vi "Synthetic_Jet_Optimisation.vi"() -> (5 "Plug in titles":string[](array[string]), 7 "Plug in values":string[](array[string]))   [LabVIEW 2011]
uses:
  Controls/SJ_Channels.ctl
  Controls/SJ_Data_Cluster.ctl
  <vilib>/Analysis/2dsp.llb/Integral Method.ctl
  Globals/Meas_global.vi
  Globals/Plug_in_data_global.vi
  <vilib>/Analysis/1siggen.llb/Ramp Pattern by Delta.vi
  <vilib>/Analysis/baseanly.llb/Scale 1D.vi
  <vilib>/Analysis/5stat.llb/RMS (DBL).vi
  <vilib>/Analysis/8numeric.llb/1D Numeric Integration.vi
  Acquisition/Data_Translation/DataTranslation_global.vi
  <vilib>/Analysis/baseanly.llb/Quick Scale 1D.vi
  <vilib>/Analysis/1siggen.llb/Ramp Pattern by Samples.vi
  <vilib>/Utility/file.llb/Write To Spreadsheet File (DBL).vi
  <vilib>/Analysis/NI_AALBase.lvlib
  <vilib>/Analysis/NI_AALPro.lvlib
panel:
  out "Target Value 2":dbl
  out "Array":dbl[][][](array[numeric])
  out "Max Amp":dbl
  out "Min Amp":dbl
  out "Sweep Frequency":dbl[](array[numeric])
  out "Last Block in Iteration?":bool
  out "Max Input Voltage _V_":dbl
  out "Sweep Size":i32
  out "Optimisation Coefficient":dbl
  out "ID Number":i32
  out "Max Number of Iterations":i32
  out "Optimisation Type":i32
  out "Target Value":dbl
  out "Phase Average?":bool
  out "Samps per cyle":i32
  out "Formation Criteria":dbl
  out "Jet Formation":bool
  out "Strouhal Number":dbl
  out "Stokes Number":dbl
  out "nu":dbl=1.55e-05
  out "Omega":dbl=1200.0
  out "Reynolds Number":dbl
  out "Charicteristic Velocity m_s":dbl
  out "Stroke Length _m_":dbl
  out "Cavity:Helmholtz:Hz":dbl=428.16291209383184
  out "LEM Velocity _ms_":dbl[](array[numeric])=[3.7049856348371377, 3.4607988115264297, 3.0653584733968287, 2.5359472607578692, 1.895702983998723, 1.1726073902466658, 0.3982632267462864, -0.3934869508418966, -1.1680398605184126, -1.8915438234131698, -2.5323782445904723, -3.062535584780142, -3.458845424238726, -3.7039871212762807, -3.787246807411894, -3.7049856348371377, -3.4607988115264297, -3.0653584733968295, -2.5359472607578692, -1.8957029839987247, -1.172607390246666, -0.3982632267462887, 0.3934869508418962, 1.1680398605184101, 1.8915438234131694, 2.53237824459047, 3.0625355847801417, 3.4588454242387248, 3.7039871212762803, 3.7872468074118935]
  out "LEM Max Velocity _ms_":dbl=3.7872475686779676
  out "LEM Phase Velocity _deg_":dbl=-258.0363282123533
  out "Phase Pressure _deg_":dbl=-169.14507601114087
  out "Phase Velocity _deg_":dbl=373.1272896341652
  out "Phase Input Voltage _deg_":dbl=8.606071626556414
  out "Phase Angle _deg_":dbl[](array[numeric])=[0.0, 12.0, 24.0, 36.0, 48.0, 60.0, 72.0, 84.0, 96.0, 108.0, 120.0, 132.0, 144.0, 156.0, 168.0, 180.0, 192.0, 204.0, 216.0, 228.0, 240.0, 252.0, 264.0, 276.0, 288.0, 300.0, 312.0, 324.0, 336.0, 348.0]
  out "Amplitude (V)":dbl=70.0
  out "Frequency (Hz)":dbl=1200.0
  out "AS Freq":dbl=36036.04
  out "Output Data Names":string[](array[string])=["Max Pressure _Pa_", "Max Velocity m_s", "Max Current _A_", "Max Displacement _m_", "Phase Displ _deg_", "Phase Pressure _deg_", "Phase Velocity _deg_", "Phase Current _deg_", "Phase Input Voltage _deg_", "LEM Max Velocity _ms_", "LEM Phase Velocity _deg_"]
  out "Input Voltage _V_":dbl[](array[numeric])=[-5.5088632433799996, -12.651031578584, -19.235618350895997, -24.9961110527, -29.670494279084004, -33.04444558276, -35.005182361704, -35.409211536216006, -34.310616683552006, -31.700640287920002, -27.711473499856005, -22.510574222680006, -16.349366000988, -9.495663135284, -2.196569584672, 5.184714435096, 12.336113665324001, 18.917564300223997, 24.689891482827996, 29.395636083331993, 32.795741589576, 34.758786092276, 35.215182844328, 34.127830748423996, 31.539748142271996, 27.582652797175996, 22.404475723135995, 16.265220463328, 9.402109185388, 2.133489422836]
  out "Pressure _Pa_":dbl[](array[numeric])=[-27.3956675953706, 95.65286233449294, 217.28142105099454, 325.3916285730047, 412.49320713856633, 477.62511872885386, 518.8812420389512, 544.5955786383588, 546.2858417945154, 525.7943338813993, 485.98446016799124, 431.53940396868336, 357.29264741860004, 257.81676584697294, 146.44897730607346, 25.39291194062997, -95.29994862668336, -216.63005998968256, -325.4638615668826, -412.65459893301875, -477.423305725176, -519.6780076017092, -543.7330519967387, -544.6659346048561, -524.568602441649, -487.2326508157636, -435.0203186855821, -361.9795522274816, -267.2741357434412, -152.01151538796677]
  out "Zeros":dbl[](array[numeric])=[1.4978743085562871, 0.2341330189017041, -0.35175473981443495, 0.0022887999999999997, -3.0068544366899315, 2.8293]
  out "Velocity m_s":dbl[](array[numeric])=[-0.006589971422005106, -0.006419643065741468, -0.009111611844261746, -0.006030326884042168, -0.004272653157727323, -0.0068849933436421745, -0.010636233235274354, -0.0035467148583991693, -0.008496862890472292, -0.005357351691532665, -0.007065956289182962, -0.006648911559621155, -0.005058171342073957, -0.008830133605031026, -0.0038751674420970687, -0.005274584307176274, 0.000979796600094568, -0.005616008146962059, -0.00729733372181674, 0.0005036149760482819, -0.004633370846616606, -0.007598533001820504, -0.005354959759266961, -0.003855515705978843, -0.005082756078867318, -0.0008163141834672163, -0.007346968606858383, -0.00413574997102441, -0.00277648312445221, -0.00052352239052674]
  out "RMS Velocity m_s":dbl=0.014914535983039488 format="%0.2f"
  out "RMS Pressure _Pa_":dbl=395.7699897259115 format="%0.2f"
  out "Max Pressure _Pa_":dbl=546.2858417945154 format="%0.2f"
  out "Max Velocity m_s":dbl=0.000979796600094568
  in  "Menu Ring":u16(ring) items=["Max Pressure _Pa_", "Input", "Max Velocity m_s"]
  out "Frequency Plot":cluster{"Sweep Frequency":dbl[], dbl[]}[](graph)
  out "Pressure Plot":cluster{dbl[], dbl[]}[](graph)=[{[0.0, 12.0, 24.0, 36.0, 48.0, 60.0, 72.0, 84.0, 96.0, 108.0, 120.0, 132.0, 144.0, 156.0, 168.0, 180.0, 192.0, 204.0, 216.0, 228.0, 240.0, 252.0, 264.0, 276.0, 288.0, 300.0, 312.0, 324.0, 336.0, 348.0], [-0.15557712257291065, -0.35728080433659803, -0.5432376920119246, -0.705921142218441, -0.8379315153272326, -0.9332160799164545, -0.9885897155857659, -1.0, -0.9689743203815658, -0.8952653536353687, -0.7826063416157439, -0.6357265029653804, -0.4617263500562873, -0.2681692905127802, -0.06203384626131485, 0.1464227586596542, 0.34838713233438734, 0.5342554516040381, 0.697273122209331, 0.8301691793748806, 0.926192371045399, 0.9816311796924717, 0.9945203893712923, 0.9638122191316959, 0.8907215601232357, 0.7789682853842954, 0.632730149899583, 0.45934997583022086, 0.26552721106968635, 0.060252384345070756]}, {[0.0, 12.0, 24.0, 36.0, 48.0, 60.0, 72.0, 84.0, 96.0, 108.0, 120.0, 132.0, 144.0, 156.0, 168.0, 180.0, 192.0, 204.0, 216.0, 228.0, 240.0, 252.0, 264.0, 276.0, 288.0, 300.0, 312.0, 324.0, 336.0, 348.0], [-0.05014896140338823, 0.1750967259562854, 0.39774309423293575, 0.5956435325215701, 0.7550867615085017, 0.8743135592895557, 0.9498346878887768, 0.9969058997564276, 1.0, 0.9624894032658751, 0.8896156974736197, 0.7899516534258018, 0.6540397353973438, 0.47194480640402603, 0.2680812243366908, 0.0464828300459258, -0.17445070206035157, -0.39655074947222896, -0.5957757581594167, -0.7553821962097238, -0.87394413180629, -0.9512932019153176, -0.9953270072140422, -0.9970346894139926, -0.9602456485390019, -0.8919005647578826, -0.7963236192550169, -0.6626193185574809, -0.4892569334498257, -0.2782636922981901]}]
  out "Velocity Plot":cluster{dbl[], dbl[]}[](graph)=[{[0.0, 12.0, 24.0, 36.0, 48.0, 60.0, 72.0, 84.0, 96.0, 108.0, 120.0, 132.0, 144.0, 156.0, 168.0, 180.0, 192.0, 204.0, 216.0, 228.0, 240.0, 252.0, 264.0, 276.0, 288.0, 300.0, 312.0, 324.0, 336.0, 348.0], [-0.15557712257291065, -0.35728080433659803, -0.5432376920119246, -0.705921142218441, -0.8379315153272326, -0.9332160799164545, -0.9885897155857659, -1.0, -0.9689743203815658, -0.8952653536353687, -0.7826063416157439, -0.6357265029653804, -0.4617263500562873, -0.2681692905127802, -0.06203384626131485, 0.1464227586596542, 0.34838713233438734, 0.5342554516040381, 0.697273122209331, 0.8301691793748806, 0.926192371045399, 0.9816311796924717, 0.9945203893712923, 0.9638122191316959, 0.8907215601232357, 0.7789682853842954, 0.632730149899583, 0.45934997583022086, 0.26552721106968635, 0.060252384345070756]}, {[0.0, 12.0, 24.0, 36.0, 48.0, 60.0, 72.0, 84.0, 96.0, 108.0, 120.0, 132.0, 144.0, 156.0, 168.0, 180.0, 192.0, 204.0, 216.0, 228.0, 240.0, 252.0, 264.0, 276.0, 288.0, 300.0, 312.0, 324.0, 336.0, 348.0], [-0.0017400427690923374, -0.0016950685794170583, -0.002405866928563968, -0.0015922719565676093, -0.001128168660507009, -0.0018179415532591603, -0.002808434141249664, -0.0009364889690996669, -0.002243546122698781, -0.0014145768585897204, -0.0018657237429983216, -0.001755605561963586, -0.0013355800662831847, -0.0023315442732039188, -0.0010232149208002786, -0.001392722622896813, 0.00025870946624789303, -0.0014828735576385352, -0.0019268175782828233, 0.00013297653986074366, -0.0012234140213805954, -0.002006347457194939, -0.0014139452830977239, -0.0010180259967302217, -0.001342071519849202, -0.00021554290622666447, -0.0019399233745421283, -0.001092020188103525, -0.0007331138596561618, -0.00013823297428152076]}, {[0.0, 12.0, 24.0, 36.0, 48.0, 60.0, 72.0, 84.0, 96.0, 108.0, 120.0, 132.0, 144.0, 156.0, 168.0, 180.0, 192.0, 204.0, 216.0, 228.0, 240.0, 252.0, 264.0, 276.0, 288.0, 300.0, 312.0, 324.0, 336.0, 348.0], [0.9782794265180274, 0.9138033477917035, 0.8093896778519208, 0.6696017951074252, 0.5005491008108334, 0.3096200089077361, 0.10515903689372944, -0.10389788964157722, -0.3084139798421589, -0.49945089918916635, -0.6686594176102914, -0.8086443108979737, -0.9132875674934984, -0.9780157749495838, -1.0, -0.9782794265180274, -0.9138033477917035, -0.8093896778519211, -0.6696017951074252, -0.5005491008108338, -0.30962000890773617, -0.10515903689373006, 0.10389788964157712, 0.3084139798421583, 0.4994508991891662, 0.6686594176102908, 0.8086443108979736, 0.9132875674934979, 0.9780157749495837, 0.9999999999999999]}]
  out "Amplitude String":string="3.5000"
  out "Frequency String":string="1200"
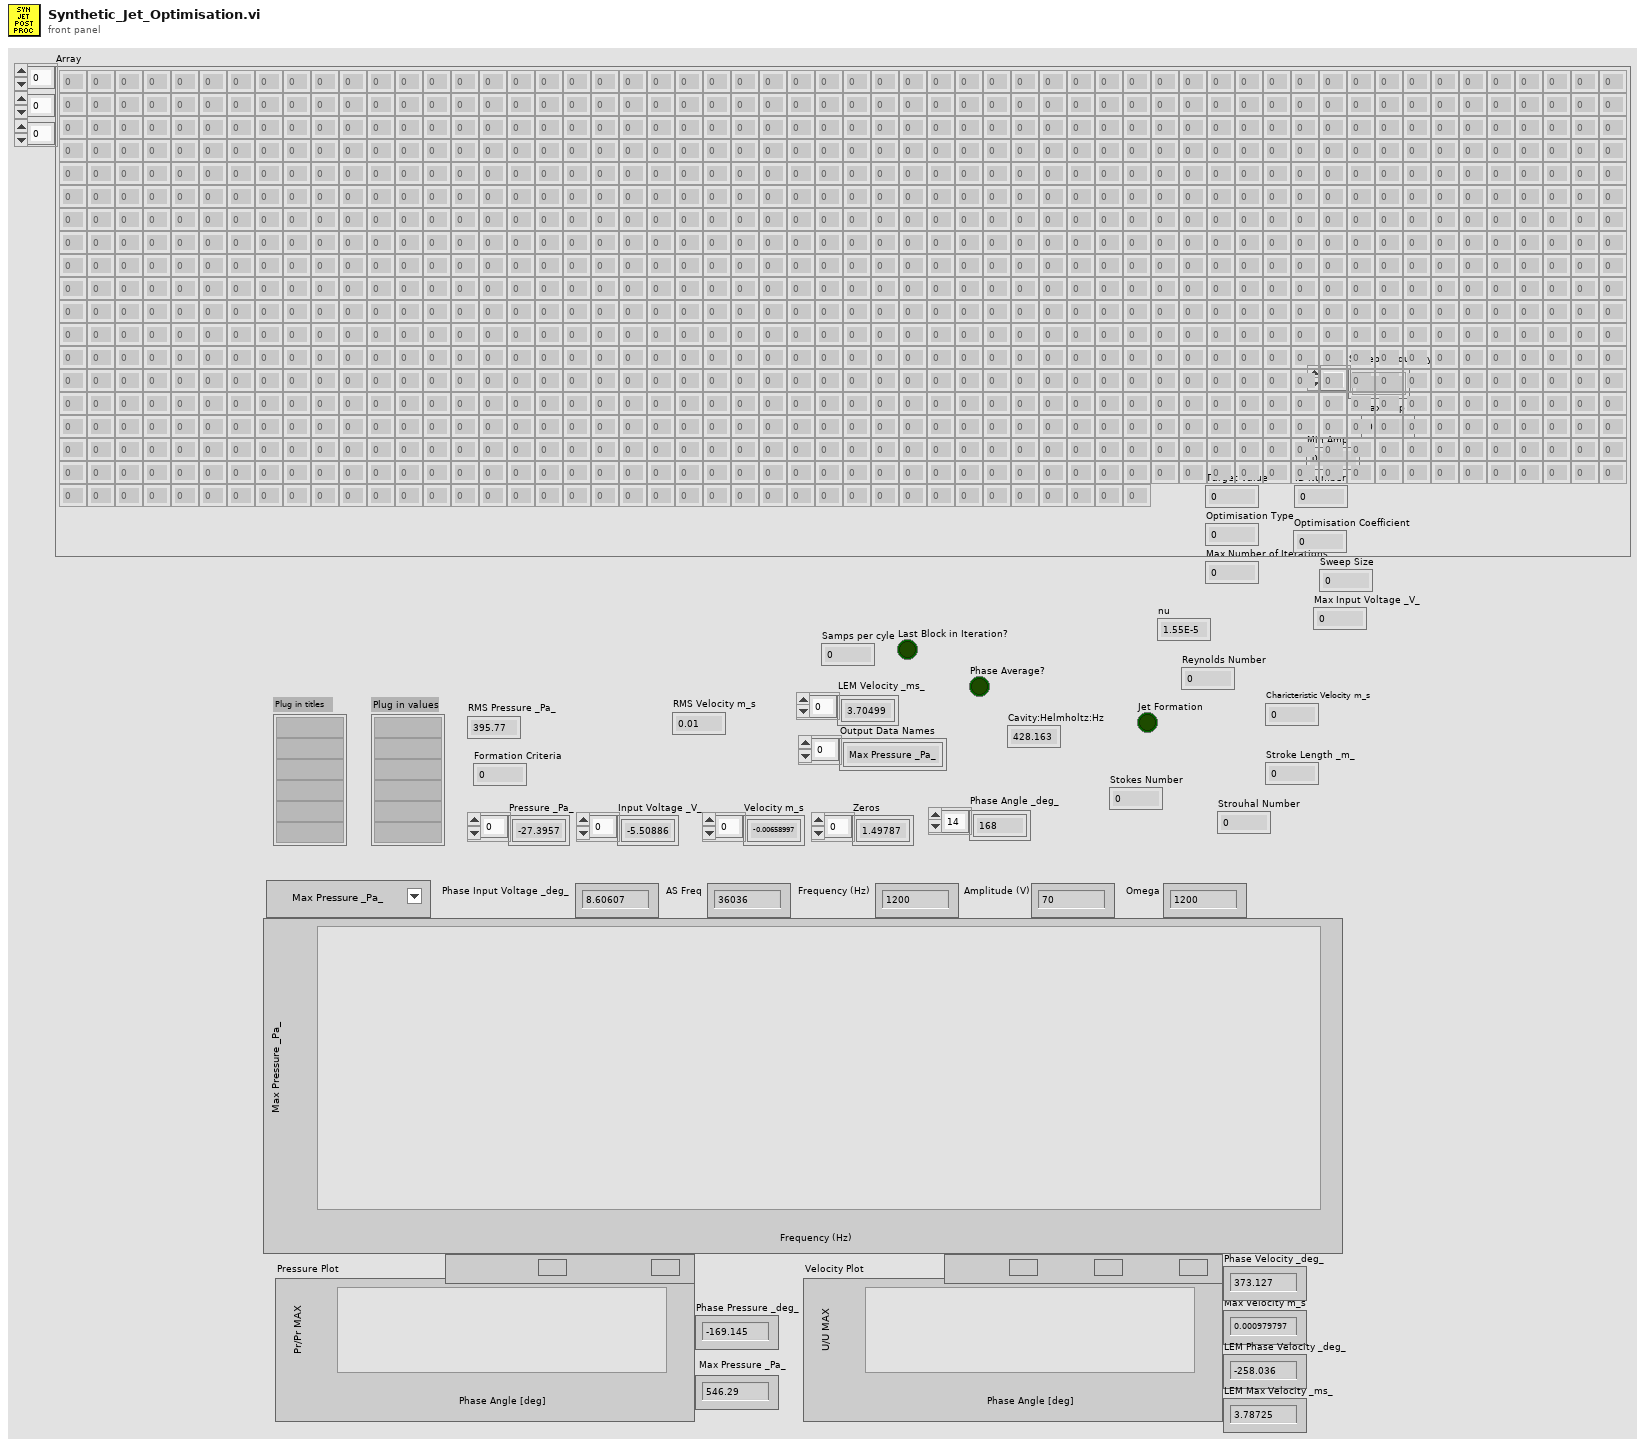
[diagram p1: front panel]
types:
  T1 = typedef "SJ_Channels.ctl" = string[]
  T2 = typedef "Analysis_info_cluster.ctl" = cluster{"Colour":u32, "Inst type":T3, "Inst name":string, "Symbol":string, "Code name":string, "Extra Info":string, "Inst Array":T4, "Index":i32, "Voltage Index":i32, "Extra Titles":string[], "Extra Values":string[]}
  T3 = typedef "Inst_type.ctl" = enum16{"Propeller anemometer", "Raw voltage", "Pressure Transducer", "Pitot-static tube", "Preston tube", "Hot wire", "Cross wire 1", "Cross wire 2", "Generic Linear", "Generic Polynomial", "Generic BackPoly", "Fast FID", "Thermocouple", "Cold wire", "Pulsed Wire", "LDA Vel", "LDA Tran time", "LDA Arr time"}
  T4 = typedef "Instrument_Array.ctl" = enum16{"PWA", "LDA", "Analogue"}
  T5 = typedef "Post_Process.ctl" = enum16{"Take New Data", "Post Process Raw Data File"}
  T6 = cluster{"Name":string, "X":dbl, "Y":dbl, "Z":dbl}[]
  T7 = typedef "SJ_Data_Cluster.ctl" = cluster{"Do":dbl, "Dc":dbl, "Ho":dbl, "Hc":dbl, "K":dbl, "beta":dbl, "Vc":dbl, "Vo":dbl}
  T8 = cluster{"R":dbl, "Mair":dbl, "T":dbl, "Patmos":dbl, "gamma":dbl}
  T9 = typedef "NI_AALPro.lvlib/Integral Method.ctl" = i32
  T10 = cluster{"Ramp Pattern":dbl[], "Y[i]=X[i]/Max|X|":dbl[]}
  T11 = cluster{"Ramp Pattern":dbl[], "Y[i]=X[i]/Max|X|":dbl[]}[]
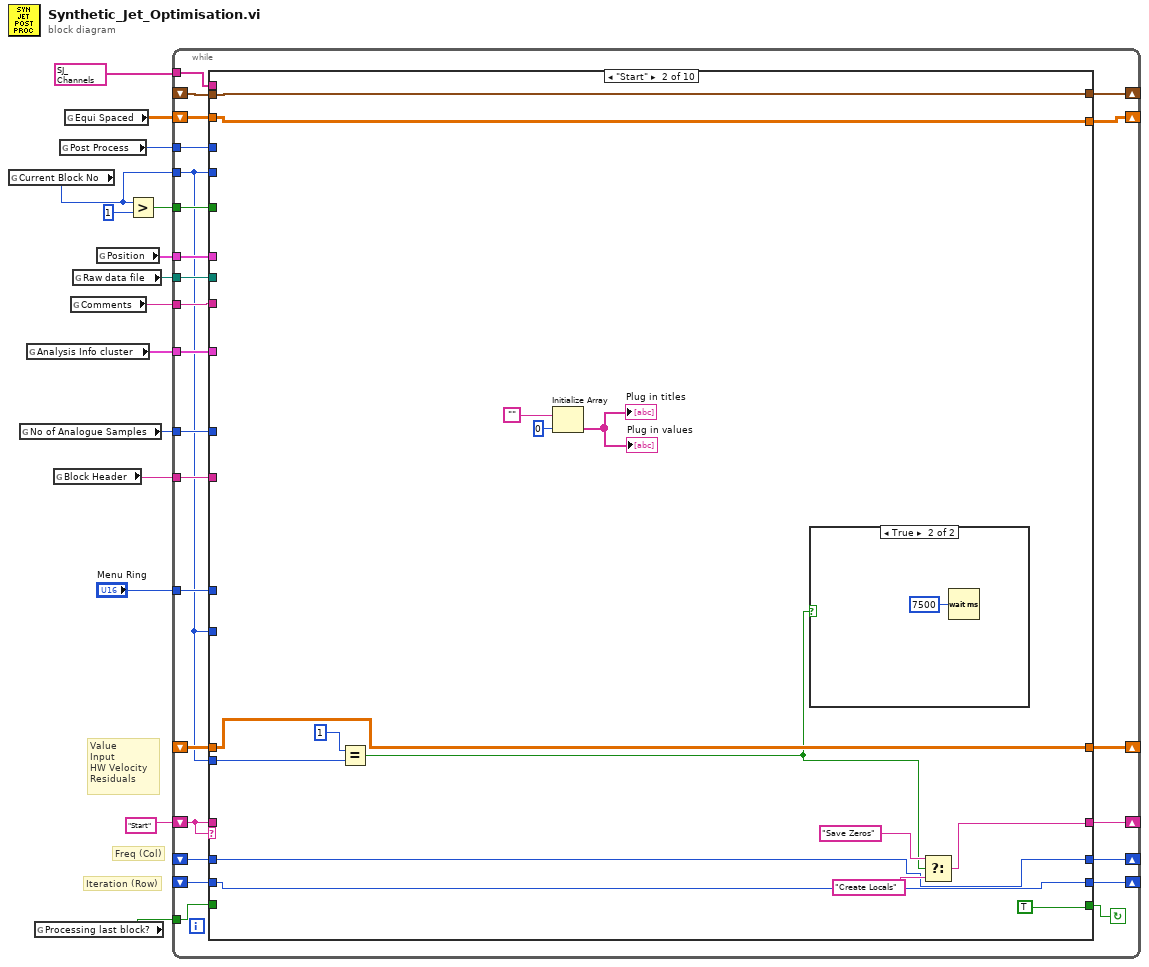
[diagram p0: block diagram]
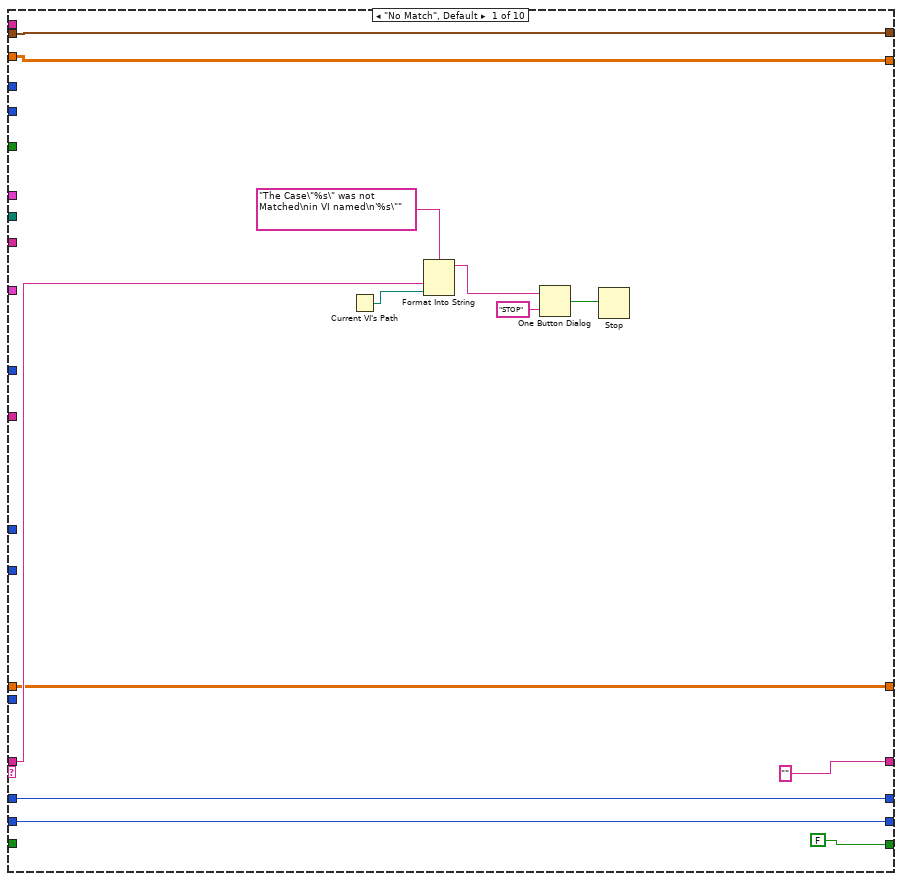
[diagram p2: hidden frame]
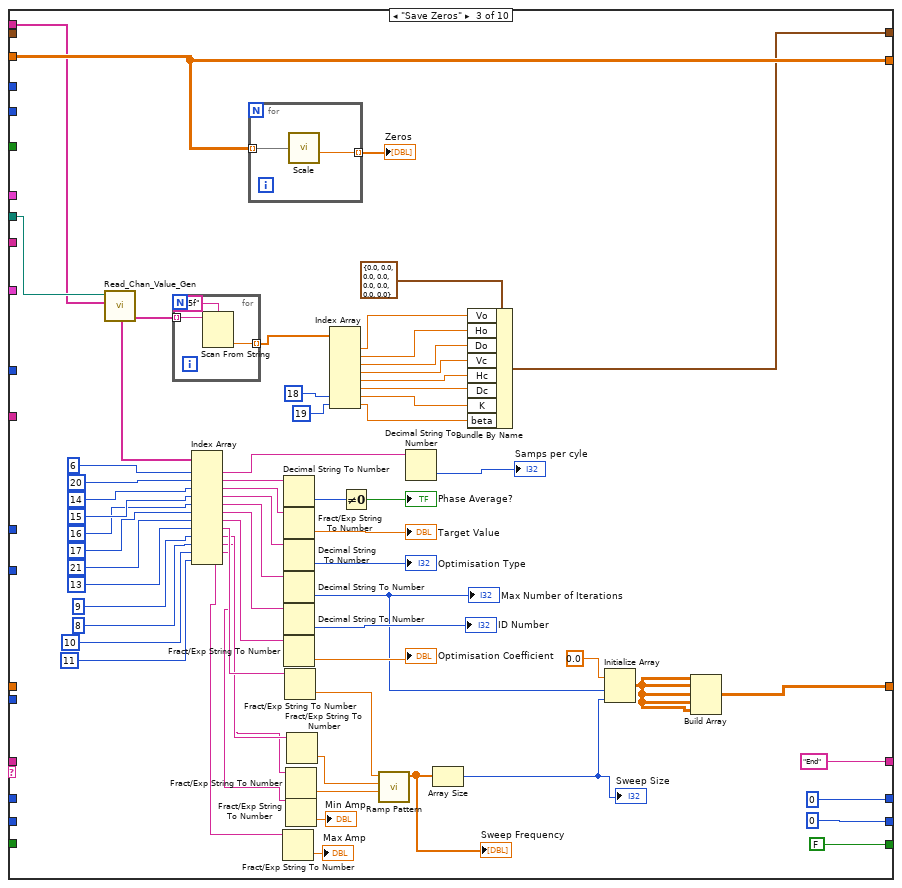
[diagram p4: hidden frame]
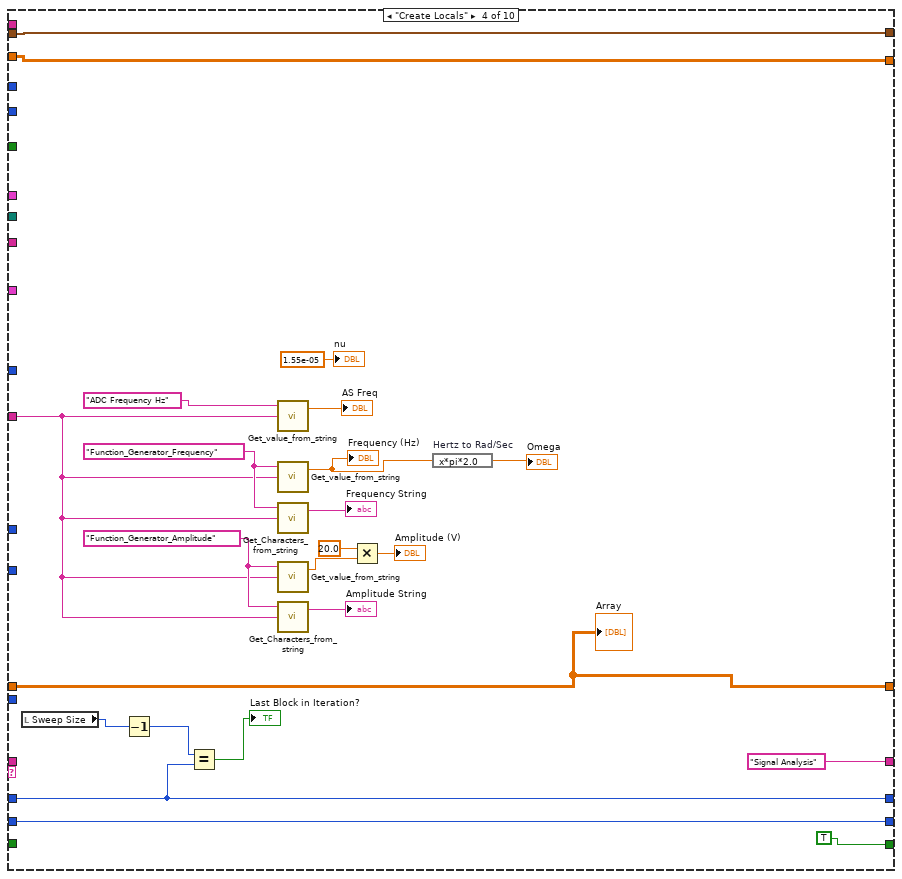
[diagram p5: hidden frame]
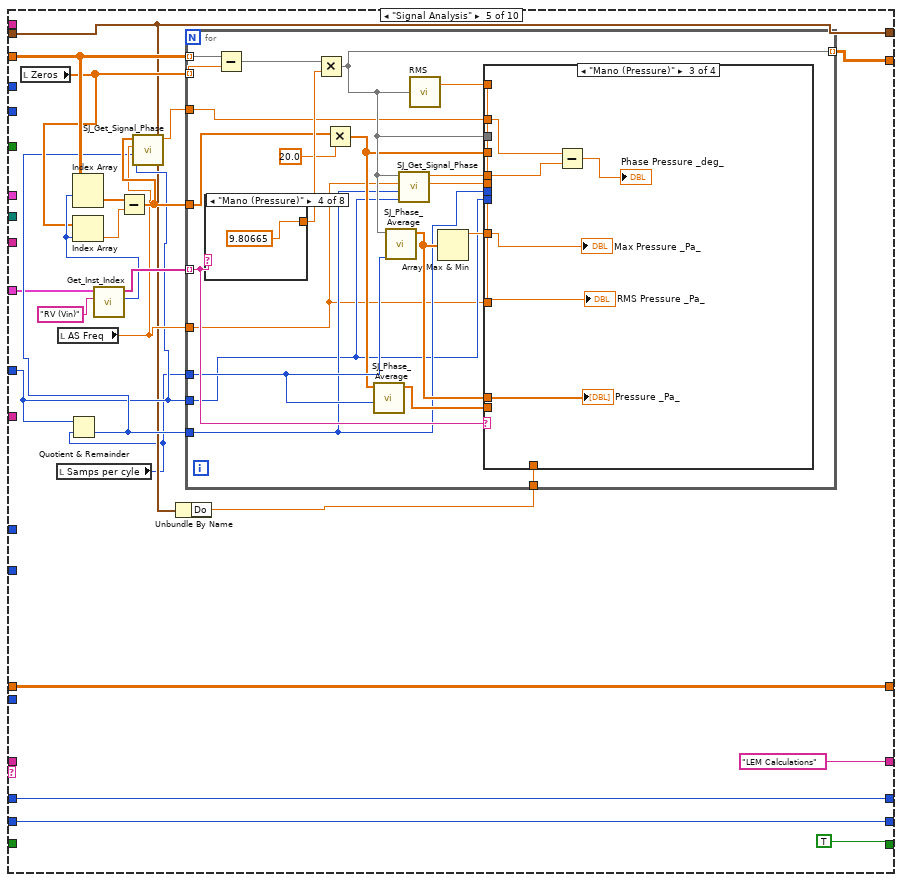
[diagram p6: hidden frame]
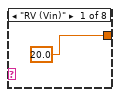
[diagram p7: hidden frame]
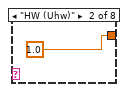
[diagram p8: hidden frame]
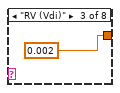
[diagram p9: hidden frame]
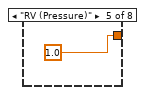
[diagram p10: hidden frame]
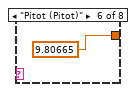
[diagram p11: hidden frame]
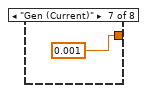
[diagram p12: hidden frame]
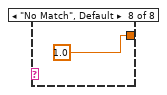
[diagram p13: hidden frame]
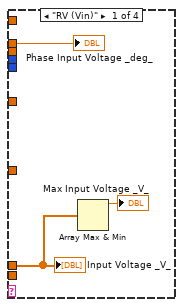
[diagram p14: hidden frame]
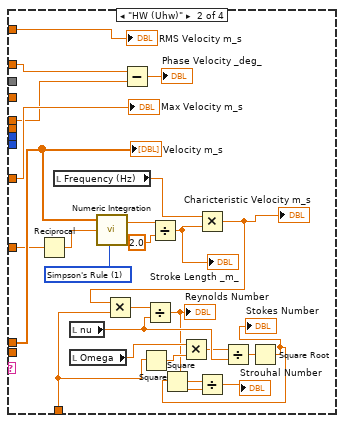
[diagram p15: hidden frame]
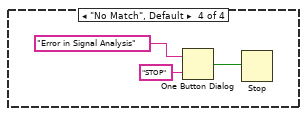
[diagram p16: hidden frame]
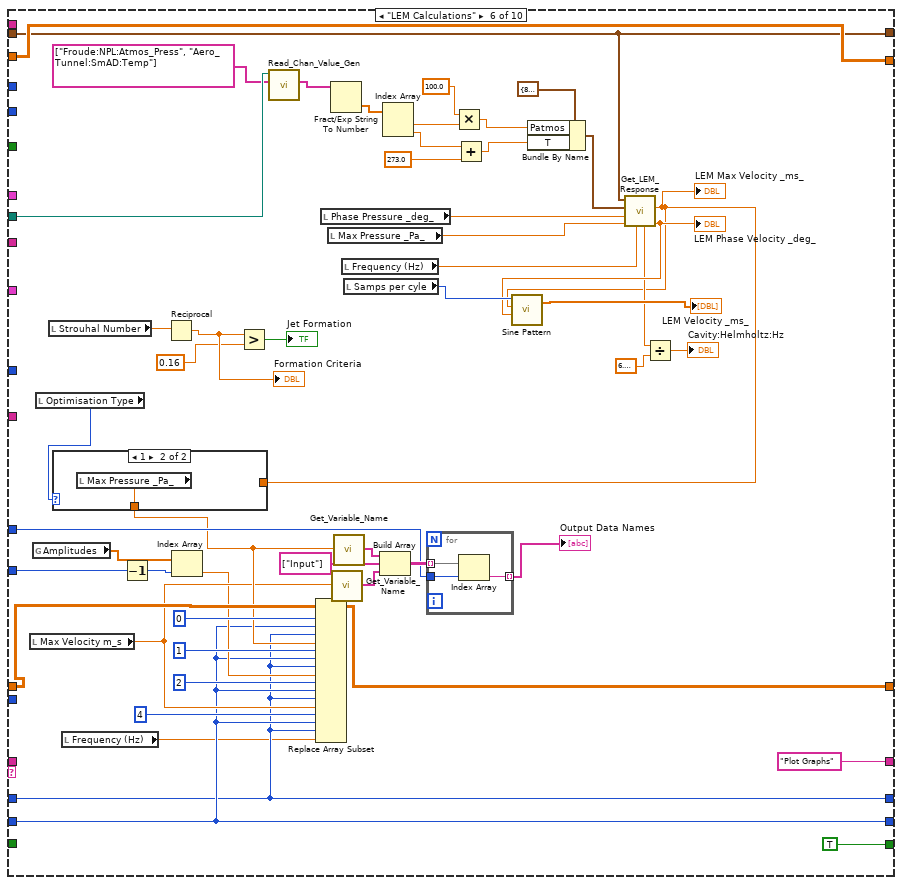
[diagram p17: hidden frame]
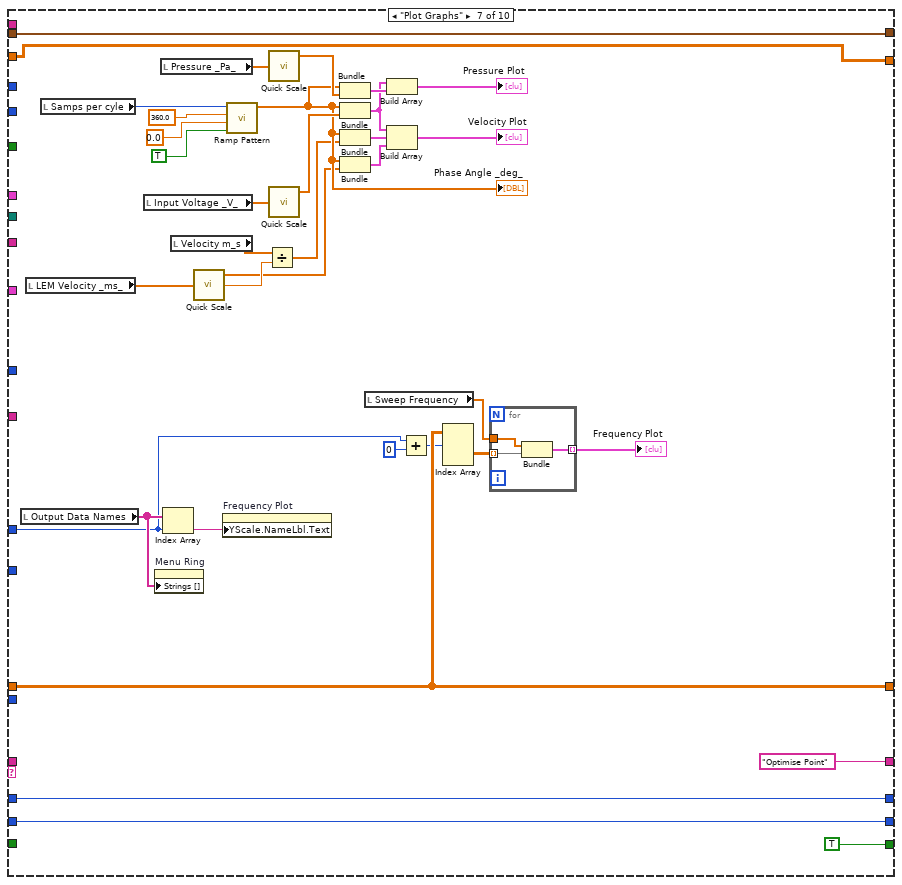
[diagram p19: hidden frame]
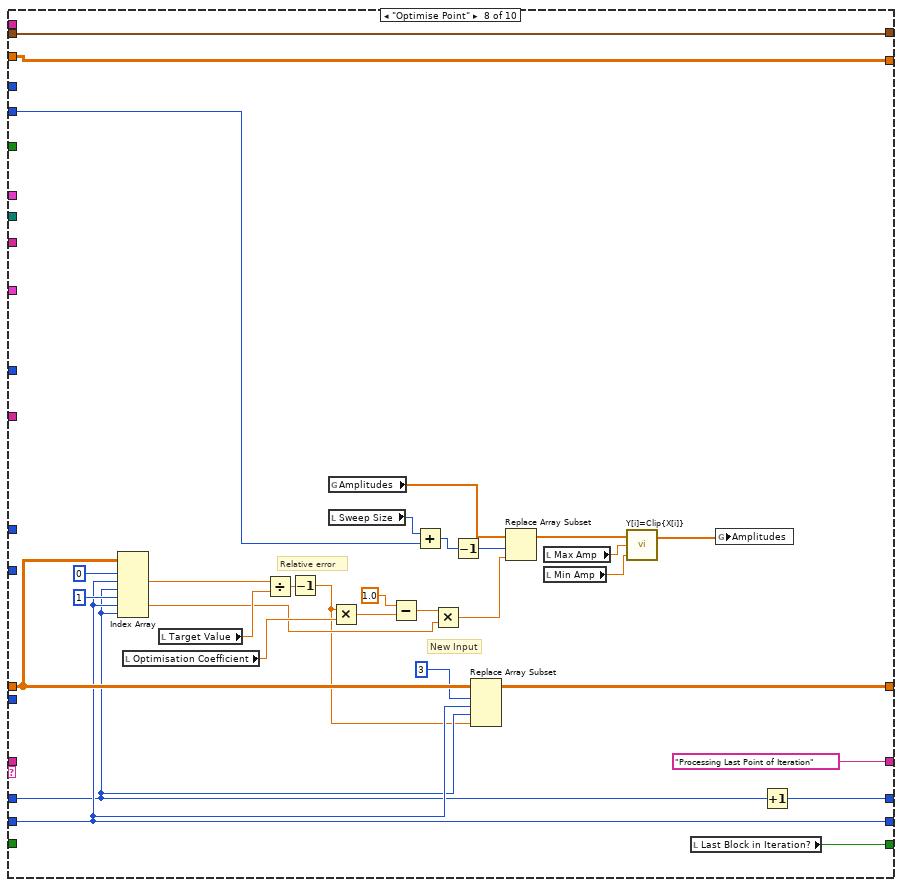
[diagram p20: hidden frame]
diagram:
  # "Iteration (Row)"
  # "Freq (Col)"
  # "Value\nInput\nHW Velocity\nResiduals"
  n1 = global read "Meas_global.vi" "Current Block No"() -> (w11:i32)
  n2 = global read "Meas_global.vi" "No of Analogue Samples"() -> (w7:i32)
  n3 = global read "Meas_global.vi" "Analysis Info cluster"() -> (w10:T2[])
  n4 = global read "Meas_global.vi" "Processing last block?"() -> (w5:bool)
  n5 = global read "Plug_in_data_global.vi" "Block Header"() -> (w8:string)
  n6 = global read "Meas_global.vi" "Post Process"() -> (w2:T5)
  n7 = global read "Plug_in_data_global.vi" "Equi Spaced"() -> (w9:dbl[][])
  n8 = global read "Meas_global.vi" "Comments"() -> (w4:string)
  n9 = global read "Meas_global.vi" "Raw data file"() -> (w14:path)
  n10 = global read "Meas_global.vi" "Position"() -> (w6:T6)
  n11 = Greater?(x=w11, y=1) -> (0:w12:bool)
  n12 = while {
    shift-left: "Start" -> [w40]
    shift-right: [w31] -> _
    tunnel: w14 -> [w39]
    tunnel: w12 -> [w38]
    tunnel: w11 -> [w16]
    tunnel: w10 -> [w37]
    tunnel: w8 -> [w35]
    tunnel: w7 -> [w34]
    tunnel: w6 -> [w33]
    tunnel: w5 -> [w32]
    shift-right: [w29] -> _
    shift-left: w9 -> [w36]
    tunnel: w4 -> [w28]
    tunnel: "Menu Ring" -> [w27]
    tunnel: w2 -> [w26]
    shift-right: [w24] -> _
    shift-left: _ -> [w25]
    tunnel: T1 ["Synthetic_Jet:Orifice:Volume", "Synthetic_Jet:Orifice:Height", "Synthetic_Jet:Orifice:Diameter", "Synthetic_Jet:Cavity:Volume", "Synthetic_Jet:Cavity:Height", "Synthetic_Jet:Cavity:Diameter", "Synthetic_Jet:Samples:Per_Cycle", "Synthetic_Jet:Dwell:Time", "Synthetic_Jet:Minimum:Frequency", "Synthetic_Jet:Maximum:Frequency", "Synthetic_Jet:Minimum:Amplitude", "Synthetic_Jet:Maximum:Amplitude", "Synthetic_Jet:Amplitude:Delta", "Synthetic_Jet:Frequency:Delta", "Synthetic_Jet:Calibration:Velocity", "Synthetic_Jet:Calibration:Type", "Synthetic_Jet:Calibration:No_Of_Gens", "Synthetic_Jet:Identification:Number", "Synthetic_Jet:LEM_Pressure:Coefficient", "Synthetic_Jet:LEM_Added_Mass:Coefficient", "Synthetic_Jet:Phase:Average?", "Synthetic_Jet:Optimisation:Coefficient"] ("Synthetic Jet Specific Channels") -> [w23]
    shift-right: [w22] -> _
    shift-left: _ -> [w21]
    shift-right: [w20] -> _
    shift-left: _ -> [w19]
    shift-right: [w18] -> _
    shift-left: _ -> [w17]
    stop <- w30 continue-if-true
    n13 = case shown="\"Start\"" w40 {
      tunnel: w40 -> [w49 _ _ _ _ _ _ _ _ _]
      tunnel: w39 -> [_ _ w127 _ _ w278 _ _ _ w383]
      tunnel: w38 -> [_ _ _ _ _ _ _ _ _ _]
      tunnel: w16 -> [_ _ _ _ _ _ _ w358 _ _]
      tunnel: w37 -> [_ _ _ _ w168 _ _ _ _ _]
      tunnel: w36 -> [w45 w59 w130 w153 w175 w297 w330 w374 w381 w406]
      tunnel: w35 -> [_ _ _ w156 _ _ _ _ _ _]
      tunnel: w34 -> [_ _ _ _ w170 _ _ _ _ _]
      tunnel: w33 -> [_ _ _ _ _ _ _ _ _ _]
      tunnel: w32 -> [_ _ _ _ _ _ _ _ w375 _]
      tunnel: w16 -> [_ w65 _ _ _ _ _ _ _ _]
      tunnel: ["" w61 "End" ("t") "Signal Analysis" "LEM Calculations" "Plot Graphs" "Optimise Point" "Processing Last Point of Iteration" ("t") "Last Block" ("t") "" ("t")] -> w31
      tunnel: [FALSE TRUE FALSE TRUE TRUE TRUE ("Processing last block?") TRUE ("Processing last block?") w371 w375 FALSE ("Processing last block?")] -> w30
      tunnel: [w45 w59 w130 w153 w181 w297 w330 w374 w381 w406] -> w29
      tunnel: w28 -> [_ _ _ _ _ _ _ _ _ _]
      tunnel: w27 -> [_ _ _ _ _ w265 w313 _ _ _]
      tunnel: w26 -> [_ _ _ _ _ _ _ _ _ _]
      tunnel: w25 -> [w44 w58 _ w145 w167 w282 w323 w373 w382 w405]
      tunnel: [w44 w58 w128 w145 w167 w282 w323 w373 w382 w405] -> w24
      tunnel: w23 -> [_ _ w126 _ _ _ _ _ _ _]
      tunnel: [w43 w56 w82 w144 w164 w261 w314 w350 w379 w384] -> w22
      tunnel: w21 -> [w43 w56 _ w144 w164 w264 w314 w355 w379 w384]
      tunnel: [w42 w57 0 ("index") w140 w163 w251 w316 w345 0 ("index") w387] -> w20
      tunnel: w19 -> [w42 w57 _ w140 w163 w251 w316 w352 _ w387]
      tunnel: [w41 w55 0 ("index") w141 w162 w252 w311 w353 w378 w404] -> w18
      tunnel: w17 -> [w41 w55 _ w141 w162 w252 w311 w353 w377 w404]
      tunnel: w16 -> [_ _ _ _ _ w256 _ _ _ _]
      frame "No Match", Default {
        n14 = Current VI's Path() -> (path=w48:path)
        n15 = Format Into String(format string="The Case\"%s\" was not Matched\nin VI named\n'%s\"" ("Format String"), w49, w48) -> (resulting string=w52:string)  [unwired: 2 in, 1 out]
        n16 = One Button Dialog(message=w52, button name ("OK")="STOP") -> (true=w50:bool)
        n17 = Stop(stop? (T)=w50) -> ()
      }
      frame "Start" {
        n18 = Equal?(x=1, y=w65) -> (x = y?=w54:bool)
        n19 = Initialize Array("", 0) -> (→"Plug in values" →"Plug in titles":string[])
        n20 = case shown="True" w54 {
          frame False {
          }
          frame True {
            n21 = Wait (ms)(milliseconds to wait=u32 7500) -> ()  [unwired: 1 out]
          }
        }
        n22 = Select(t="Save Zeros", s=w54, f="Create Locals") -> (s? t:f=w61:string)
      }
      frame "Save Zeros" {
        (unwired) FALSE ("Processing last block?")
        (unwired) "End" ("t")
        (unwired) "End" ("t")
        (unwired) FALSE ("Processing last block?")
        n23 = call "Read_Chan_Value_Gen.vi"("Desired Ch Names"=w126, "Raw data file"=w127) -> ("Values"=w106:string[])  [unwired: 9 in]
        n24 = for {
          tunnel: w106 -> [w136] mode=indexing
          tunnel: [w134] -> w115 mode=indexing
          n25 = Scan From String(format string="%5f", input string=w136) -> (output 1=w134:dbl)  [unwired: 3 in, 3 out]
        }
        n26 = Index Array(array=w106, index #1=6 ("index"), index #2=20 ("index"), index #3=14 ("index"), index #4=15 ("index"), index #5=16 ("index"), index #6=17 ("index"), index #7=21 ("index"), index #8=13 ("index"), index #9=9 ("index"), index #10=8 ("index"), index #11=10 ("index"), index #12=11 ("index")) -> (element #1=w113:string, element #2=w105:string, element #3=w104:string, element #4=w103:string, element #5=w102:string, element #6=w101:string, element #7=w100:string, element #8=w90:string, element #9=w89:string, element #10=w88:string, element #11=w79:string, element #12=w78:string)
        n27 = for {
          tunnel: w130 -> [w138] mode=indexing
          tunnel: [w137] -> w132 mode=indexing
          n28 = call-poly <vilib>:"Scale.vi"("X"=w138) -> ("offset"=w137:dbl)  [unwired: 3 out]
        }
        "Zeros" <- w132
        n29 = Fract/Exp String To Number(string=w78) -> (number=→"Max Amp":dbl)  [unwired: 3 in, 1 out]
        n30 = Decimal String To Number(string=w105) -> (number=w111:i32)  [unwired: 2 in, 1 out]
        n31 = Fract/Exp String To Number(string=w104) -> (number=→"Target Value":dbl)  [unwired: 3 in, 1 out]
        n32 = Decimal String To Number(string=w103) -> (number=→"Optimisation Type":i32)  [unwired: 2 in, 1 out]
        n33 = Decimal String To Number(string=w102) -> (number=w73:i32)  [unwired: 2 in, 1 out]
        "Max Number of Iterations" <- w73
        n34 = Decimal String To Number(string=w101) -> (number=→"ID Number":i32)  [unwired: 2 in, 1 out]
        n35 = Fract/Exp String To Number(string=w100) -> (number=→"Optimisation Coefficient":dbl)  [unwired: 3 in, 1 out]
        n36 = Fract/Exp String To Number(string=w90) -> (number=w87:dbl)  [unwired: 3 in, 1 out]
        n37 = Fract/Exp String To Number(string=w88) -> (number=w85:dbl)  [unwired: 3 in, 1 out]
        n38 = Fract/Exp String To Number(string=w79) -> (number=→"Min Amp":dbl)  [unwired: 3 in, 1 out]
        n39 = Fract/Exp String To Number(string=w89) -> (number=w86:dbl)  [unwired: 3 in, 1 out]
        n40 = Index Array(array=w115, index #7=18 ("index"), index #8=19 ("index")) -> (element #1=w125:dbl, element #2=w124:dbl, element #3=w123:dbl, element #4=w122:dbl, element #5=w121:dbl, element #6=w120:dbl, element #7=w117:dbl, element #8=w116:dbl)  [unwired: 6 in]
        n41 = Not Equal To 0?(x=w111) -> (x != 0?=→"Phase Average?":bool)
        n42 = call-poly <vilib>:"Ramp Pattern.vi"("start"=w85, "end"=w86, "delta"=w87) -> ("Ramp Pattern"=w84:dbl[])  [unwired: 6 in, 2 out]
        "Sweep Frequency" <- w84
        n43 = Decimal String To Number(string=w113) -> (number=→"Samps per cyle":i32)  [unwired: 2 in, 1 out]
        n44 = Array Size(array=w84) -> (size(s)=w74:i32)
        "Sweep Size" <- w74
        n45 = Bundle By Name(cluster=T7 {"Do"=0.0, "Dc"=0.0, "Ho"=0.0, "Hc"=0.0, "K"=0.0, "beta"=0.0, "Vc"=0.0, "Vo"=0.0} ("SJ_Data_Cluster"), "Vo"=w125, "Ho"=w124, "Do"=w123, "Vc"=w122, "Hc"=w121, "Dc"=w120, "K"=w117, "beta"=w116) -> (w128:T7)
        n46 = Initialize Array(0.0 ("element"), w73, w74) -> (w70:dbl[][])
        n47 = Build Array(w70, w70, w70, w70, w70) -> (w82:dbl[][][])
      }
      frame "Create Locals" {
        w158 = "Function_Generator_Amplitude" ("Variable name")
        w159 = "Function_Generator_Frequency" ("Variable name")
        n48 = local read "Sweep Size"() -> (w143:i32)
        n49 = Decrement(x=w143) -> (x-1=w142:i32)
        n50 = Equal?(x=w142, y=w140) -> (x = y?=→"Last Block in Iteration?":bool)
        n51 = call "Get_value_from_string.vi"("Input string"=w156, "Variable name"="ADC Frequency Hz") -> ("Value"=→"AS Freq":dbl)  [unwired: 1 in, 1 out]
        n52 = call "Get_value_from_string.vi"("Input string"=w156, "Variable name"=w159) -> ("Value"=w148:dbl)  [unwired: 1 in, 1 out]
        "Frequency (Hz)" <- w148
        n53 = call "Get_Characters_from_string.vi"("Input string"=w156, "Variable name"=w159) -> ("Value"=→"Frequency String":string)  [unwired: 1 in, 1 out]
        n54 = call "Get_value_from_string.vi"("Input string"=w156, "Variable name"=w158) -> ("Value"=w151:dbl)  [unwired: 1 in, 1 out]
        n55 = call "Get_Characters_from_string.vi"("Input string"=w156, "Variable name"=w158) -> ("Value"=→"Amplitude String":string)  [unwired: 1 in, 1 out]
        n56 = Multiply(x=20.0, y=w151) -> (x*y=→"Amplitude (V)":dbl)
        n57 = expression code="x*pi*2.0" "Hertz to Rad/Sec"(w148) -> (→"Omega":dbl)
        "nu" <- 1.55e-05 ("y")
        "Array" <- w144
      }
      frame "Signal Analysis" {
        n58 = local read "Zeros"() -> (w174:dbl[])
        n59 = local read "Samps per cyle"() -> (w165:i32)
        n60 = local read "AS Freq"() -> (w172:dbl)
        n61 = Quotient & Remainder(x=w170, y=w165) -> (floor(x/y)=w171:i32)  [unwired: 1 out]
        n62 = call "Get_Inst_Index.vi"("Inst name search"="RV (Vin)" ("element"), "Analysis Info cluster"=w168) -> ("Index of Instance"=w176:i32, "Inst Name Array"=w179:string[])  [unwired: 7 in, 1 out]
        n63 = Index Array(array=w175, index (row)=w176) -> (element=w177:dbl[])  [unwired: 1 in]
        n64 = Index Array(array=w174, index=w176) -> (element=w178:dbl)
        n65 = Subtract(x=w177, y=w178) -> (x-y=w173:dbl[])
        n66 = call "SJ_Get_Signal_Phase.vi"("No of Analogue Samples"=w170, "Number of Cycles"=w171, "Actual Sampling Frequency"=w172, "Signal"=w173) -> ("Phase Angle _deg_"=w169:dbl)  [unwired: 7 in]
        n67 = Unbundle By Name(w167) -> ("Do"=w166:dbl)
        n68 = for {
          tunnel: w175 -> [w203] mode=indexing
          tunnel: w174 -> [w202] mode=indexing
          tunnel: [w191] -> w181 mode=indexing
          tunnel: w179 -> [w200] mode=indexing
          tunnel: w165 -> [w193]
          tunnel: w172 -> [w185]
          tunnel: w170 -> [w188]
          tunnel: w171 -> [w189]
          tunnel: w173 -> [w187]
          tunnel: w169 -> [w186]
          tunnel: w166 -> [w184]
          n69 = case shown="\"Mano (Pressure)\"" w200 {
            tunnel: [20.0 1.0 0.002 9.80665 1.0 9.80665 0.001 1.0] -> w198
            frame "RV (Vin)" {
            }
            frame "HW (Uhw)" {
            }
            frame "RV (Vdi)" {
            }
            frame "Mano (Pressure)" {
            }
            frame "RV (Pressure)" {
            }
            frame "Pitot (Pitot)" {
            }
            frame "Gen (Current)" {
            }
            frame "No Match", Default {
            }
          }
          n70 = Subtract(x=w203, y=w202) -> (x-y=w201:dbl[])
          n71 = Multiply(x=w201, y=w198) -> (x*y=w191:dbl[])
          n72 = Multiply(x=w187, y=20.0) -> (x*y=w190:dbl[])
          n73 = call "SJ_Phase_Average.vi"("No. of Bins"=w193, "1D Signal"=w190) -> ("Phase Averaged Signal"=w196:dbl[])  [unwired: 7 in, 2 out]
          n74 = call "SJ_Phase_Average.vi"("No. of Bins"=w193, "1D Signal"=w191) -> ("Phase Averaged Signal"=w195:dbl[])  [unwired: 7 in, 2 out]
          n75 = call "SJ_Get_Signal_Phase.vi"("No of Analogue Samples"=w188, "Number of Cycles"=w189, "Actual Sampling Frequency"=w185, "Signal"=w191) -> ("Phase Angle _deg_"=w192:dbl)  [unwired: 7 in]
          n76 = call-poly <vilib>:"RMS.vi"("X"=w191) -> ("rms value"=w199:dbl)  [unwired: 1 out]
          n77 = Array Max & Min(array=w195) -> (max value=w194:dbl)  [unwired: 3 out]
          n78 = case shown="\"Mano (Pressure)\"" w200 {
            tunnel: w195 -> [w213 w234 w245 _]
            tunnel: w196 -> [_ _ _ _]
            tunnel: w199 -> [_ w239 w244 _]
            tunnel: w194 -> [_ w238 w243 _]
            tunnel: w192 -> [w214 w237 w241 _]
            tunnel: w191 -> [_ _ _ _]
            tunnel: w190 -> [_ _ _ _]
            tunnel: w185 -> [_ _ _ _]
            tunnel: w189 -> [_ _ _ _]
            tunnel: w188 -> [_ _ _ _]
            tunnel: w186 -> [_ w236 w242 _]
            tunnel: w185 -> [_ w232 _ _]
            tunnel: w184 -> [_ w223 _ _]
            frame "RV (Vin)" {
              n79 = Array Max & Min(array=w213) -> (max value=→"Max Input Voltage _V_":dbl)  [unwired: 3 out]
              "Input Voltage _V_" <- w213
              "Phase Input Voltage _deg_" <- w214
            }
            frame "HW (Uhw)" {
              w233 = T9 1 items=["Trapezoidal Rule", "Simpson's Rule", "Simpson's 3/8 Rule", "Bode Rule"] ("integration method")
              n80 = Reciprocal(x=w232) -> (1/x=w231:dbl)
              n81 = local read "Frequency (Hz)"() -> (w227:dbl)
              n82 = local read "nu"() -> (w221:dbl)
              n83 = local read "Omega"() -> (w222:dbl)
              n84 = call-poly <vilib>:"Numeric Integration.vi"("integration method"=w233, "dt"=w231, "Input Array"=w234) -> ("result"=w230:dbl)  [unwired: 1 out]
              n85 = Subtract(x=w236, y=w237) -> (x-y=→"Phase Velocity _deg_":dbl)
              n86 = Square(x=w223) -> (x^2=w224:dbl)
              n87 = Divide(x=w230, y=2.0) -> (x/y=w228:dbl)
              "Stroke Length _m_" <- w228
              n88 = Multiply(x=w222, y=w224) -> (x*y=w220:dbl)
              n89 = Multiply(x=w227, y=w228) -> (x*y=w226:dbl)
              "Charicteristic Velocity m_s" <- w226
              n90 = Multiply(x=w226, y=w223) -> (x*y=w225:dbl)
              n91 = Divide(x=w225, y=w221) -> (x/y=w218:dbl)
              "Reynolds Number" <- w218
              n92 = Divide(x=w220, y=w221) -> (x/y=w219:dbl)
              n93 = Square Root(x=w219) -> (sqrt(x)=w216:dbl)
              "Stokes Number" <- w216
              n94 = Square(x=w216) -> (x^2=w217:dbl)
              n95 = Divide(x=w217, y=w218) -> (x/y=→"Strouhal Number":dbl)
              "Velocity m_s" <- w234
              "RMS Velocity m_s" <- w239
              "Max Velocity m_s" <- w238
            }
            frame "Mano (Pressure)" {
              n96 = Subtract(x=w242, y=w241) -> (x-y=→"Phase Pressure _deg_":dbl)
              "Pressure _Pa_" <- w245
              "RMS Pressure _Pa_" <- w244
              "Max Pressure _Pa_" <- w243
            }
            frame "No Match", Default {
              n97 = One Button Dialog(message="Error in Signal Analysis", button name ("OK")="STOP") -> (true=w247:bool)
              n98 = Stop(stop? (T)=w247) -> ()
            }
          }
        }
      }
      frame "LEM Calculations" {
        n99 = local read "Max Velocity m_s"() -> (w258:dbl)
        n100 = global read "DataTranslation_global.vi" "Amplitudes"() -> (w257:dbl[])
        n101 = local read "Optimisation Type"() -> (w271:i32)
        n102 = local read "Strouhal Number"() -> (w275:dbl)
        n103 = local read "Frequency (Hz)"() -> (w250:dbl)
        n104 = Decrement(x=w256) -> (x-1=w254:i32)
        n105 = Reciprocal(x=w275) -> (1/x=w274:dbl)
        "Formation Criteria" <- w274
        n106 = Index Array(array=w257, index=w254) -> (element=w255:dbl)
        n107 = Greater?(x=w274, y=0.16) -> (0:→"Jet Formation":bool)
        n108 = call "Read_Chan_Value_Gen.vi"("Desired Ch Names"=string[] ["Froude:NPL:Atmos_Press", "Aero_Tunnel:SmAD:Temp"], "Raw data file"=w278) -> ("Values"=w276:string[])  [unwired: 9 in]
        n109 = local read "Phase Pressure _deg_"() -> (w287:dbl)
        n110 = local read "Max Pressure _Pa_"() -> (w288:dbl)
        n111 = Fract/Exp String To Number(string=w276) -> (number=w296:dbl[])  [unwired: 3 in, 1 out]
        n112 = call "Get_Variable_Name.vi"("Data"=w258) -> ("Data Name(s)"=w269:string[])  [unwired: 24 in, 2 out]
        n113 = local read "Frequency (Hz)"() -> (w286:dbl)
        n114 = local read "Samps per cyle"() -> (w285:i32)
        n115 = Index Array(array=w296) -> (element #1=w293:dbl, element #2=w295:dbl)  [unwired: 2 in]
        n116 = Multiply(x=100.0 ("y"), y=w293) -> (x*y=w291:dbl)
        n117 = Add(x=w295, y=273.0) -> (x+y=w294:dbl)
        n118 = Bundle By Name(cluster=T8 {"R"=8.31451, "Mair"=0.0289645, "T"=293.0, "Patmos"=101325.0, "gamma"=1.4} ("Fluid Properties"), "Patmos"=w291, "T"=w294) -> (w289:T8)
        n119 = call "Get_LEM_Response.vi"("Frequency (Hz)"=w286, "Cavity Pressure Magnitude"=w288, "Cavity Pressure Phase"=w287, "Fluid Properties"=w289, "SJ Data IN"=w282) -> ("Phi"=w284:dbl, "Uo"=w270:dbl, "OmegaH"=w281:dbl)  [unwired: 2 in, 2 out]
        "LEM Phase Velocity _deg_" <- w284
        "LEM Max Velocity _ms_" <- w270
        n120 = case shown="1" w271 {
          tunnel: w270 -> [w304 _]
          tunnel: [w304 w305] -> w260
          frame 0, Default {
          }
          frame 1 {
            n121 = local read "Max Pressure _Pa_"() -> (w305:dbl)
          }
        }
        n122 = Replace Array Subset(array=w264, new element #1=w260, index (dim 0) #1=0 ("index (page)"), index (dim 1) #1=w252, index (dim 2) #1=w251, new element #2=w255, index (dim 0) #2=1 ("index (page)"), index (dim 1) #2=w252, index (dim 2) #2=w251, new element #3=w258, index (dim 0) #3=2 ("index (page)"), index (dim 1) #3=w252, index (dim 2) #3=w251, new element #4=w250, index (dim 0) #4=4 ("index (page)"), index (dim 1) #4=w252, index (dim 2) #4=w251) -> (w261:dbl[][][])
        n123 = call "Get_Variable_Name.vi"("Data"=w260) -> ("Data Name(s)"=w268:string[])  [unwired: 24 in, 2 out]
        n124 = Build Array(w268, string[] ["Input"] ("element"), w269) -> (w267:string[][])
        n125 = for {
          tunnel: w267 -> [w303] mode=indexing
          tunnel: [w302] -> w266 mode=indexing
          tunnel: w265 -> [w301]
          n126 = Index Array(array=w303, index=w301) -> (element=w302:string)
        }
        "Output Data Names" <- w266
        n127 = call <vilib>:"Sine Pattern.vi"("phase(degrees)"=w284, "amplitude"=w270, "samples"=w285) -> ("Sinusoidal Pattern"=→"LEM Velocity _ms_":dbl[])  [unwired: 1 in, 1 out]
        n128 = Divide(x=w281, y=6.283185307179586) -> (x/y=→"Cavity:Helmholtz:Hz":dbl)
      }
      frame "Plot Graphs" {
        n129 = local read "Output Data Names"() -> (w315:string[])
        n130 = local read "LEM Velocity _ms_"() -> (w321:dbl[])
        n131 = local read "Samps per cyle"() -> (w333:i32)
        n132 = local read "Input Voltage _V_"() -> (w329:dbl[])
        n133 = property on="Menu Ring" class="Ring (strict)"("Strings []"=w315) -> ()  [unwired: 2 in, 2 out]
        n134 = local read "Pressure _Pa_"() -> (w327:dbl[])
        n135 = Index Array(array=w315, index=w313) -> (element=w334:string)
        n136 = local read "Velocity m_s"() -> (w318:dbl[])
        n137 = call-poly <vilib>:"Quick Scale.vi"("X"=w321) -> ("Y[i]=X[i]/Max|X|"=w319:dbl[], "max|X|"=w320:dbl)  [unwired: 1 out]
        n138 = property on="Frequency Plot" class="XYGraph (strict)"("YScale.NameLbl.Text"=w334) -> ()  [unwired: 2 in, 2 out]
        n139 = call-poly <vilib>:"Ramp Pattern.vi"("exclude end?"=TRUE, "start"=0.0, "end"=360.0, "samples"=w333) -> ("Ramp Pattern"=w324:dbl[])  [unwired: 6 in, 1 out]
        "Phase Angle _deg_" <- w324
        n140 = Divide(x=w318, y=w320) -> (x/y=w317:dbl[])
        n141 = call-poly <vilib>:"Quick Scale.vi"("X"=w327) -> ("Y[i]=X[i]/Max|X|"=w326:dbl[])  [unwired: 2 out]
        n142 = call-poly <vilib>:"Quick Scale.vi"("X"=w329) -> ("Y[i]=X[i]/Max|X|"=w328:dbl[])  [unwired: 2 out]
        n143 = Bundle("Ramp Pattern"=w324, "Y[i]=X[i]/Max|X|"=w326) -> (w338:T10)  [unwired: 1 in]
        n144 = Bundle("Ramp Pattern"=w324, "Y[i]=X[i]/Max|X|"=w328) -> (w335:T10)  [unwired: 1 in]
        n145 = Bundle("Ramp Pattern"=w324, w317) -> (w339:cluster{"Ramp Pattern":dbl[], dbl[]})  [unwired: 1 in]
        n146 = Bundle("Ramp Pattern"=w324, "Y[i]=X[i]/Max|X|"=w319) -> (w325:T10)  [unwired: 1 in]
        n147 = local read "Sweep Frequency"() -> (w312:dbl[])
        n148 = Build Array(w335, w338) -> (→"Pressure Plot":T11)
        n149 = Build Array(w335, w339, w325) -> (→"Velocity Plot":T11)
        n150 = Add(x=w313, y=u16 0) -> (x+y=w310:u16)
        n151 = Index Array(array=w314, index (dim 0)=w310) -> (element=w308:dbl[][])  [unwired: 2 in]
        n152 = for {
          tunnel: w312 -> [w343]
          tunnel: w308 -> [w342] mode=indexing
          tunnel: [w341] -> w307 mode=indexing
          n153 = Bundle("Sweep Frequency"=w343, w342) -> (w341:cluster{"Sweep Frequency":dbl[], dbl[]})  [unwired: 1 in]
        }
        "Frequency Plot" <- w307
      }
      frame "Optimise Point" {
        # "New Input"
        # "Relative error"
        n154 = Index Array(array=w355, index (dim 0) #1=0 ("index (page)"), index (dim 1) #1=w353, index (dim 2) #1=w352, index (dim 0) #2=1 ("index (page)"), index (dim 1) #2=w353, index (dim 2) #2=w352) -> (element #1=w368:dbl, element #2=w361:dbl)
        n155 = local read "Optimisation Coefficient"() -> (w365:dbl)
        n156 = local read "Target Value"() -> (w367:dbl)
        n157 = Divide(x=w368, y=w367) -> (x/y=w366:dbl)
        n158 = Decrement(x=w366) -> (x-1=w351:dbl)
        n159 = global read "DataTranslation_global.vi" "Amplitudes"() -> (w360:dbl[])
        n160 = local read "Sweep Size"() -> (w359:i32)
        n161 = Multiply(x=w351, y=w365) -> (x*y=w364:dbl)
        n162 = Subtract(x=1.0, y=w364) -> (x-y=w362:dbl)
        n163 = Add(x=w359, y=w358) -> (x+y=w357:i32)
        n164 = Multiply(x=w362, y=w361) -> (x*y=w356:dbl)
        n165 = Decrement(x=w357) -> (x-1=w346:i32)
        n166 = Replace Array Subset(array=w355, new element=w351, index (dim 0)=3 ("index (page)"), index (dim 1)=w353, index (dim 2)=w352) -> (w350:dbl[][][])
        n167 = Replace Array Subset(array=w360, new element=w356, index=w346) -> (w349:dbl[])
        n168 = local read "Max Amp"() -> (w348:dbl)
        n169 = local read "Min Amp"() -> (w347:dbl)
        n170 = call <vilib>:"Y[i]=Clip{X[i]}.vi"("lower limit"=w347, "upper limit"=w348, "Input Array"=w349) -> ("Clipped Array"=w344:dbl[])  [unwired: 1 out]
        n171 = local read "Last Block in Iteration?"() -> (w371:bool)
        n172 = global write "DataTranslation_global.vi" "Amplitudes"(w344) -> ()
        n173 = Increment(x=w352) -> (x+1=w345:i32)
      }
      frame "Processing Last Point of Iteration" {
        n174 = Increment(x=w377) -> (x+1=w378:i32)
      }
      frame "Last Block" {
        n175 = Strip Path(path=w383) -> (stripped path=w399:path)  [unwired: 1 out]
        n176 = local read "Target Value 2"() -> (w393:dbl)
        n177 = Strip Path(path=w399) -> (stripped path=w401:path, name=w395:string)
        n178 = Strip Path(path=w401) -> (stripped path=w400:path)  [unwired: 1 out]
        n179 = Strip Path(path=w400) -> (stripped path=w402:path)  [unwired: 1 out]
        n180 = Build Path(base path=w402, name or relative path="Results_Post_Processed") -> (appended path=w398:path)
        n181 = Number To Fractional String(number=w393, width (-)=i16 3 ("precision (6)"), precision (6)=i16 0) -> (F-format string=w391:string)  [unwired: 1 in]
        n182 = Build Path(base path=w398, name or relative path="Optimisation" ("New Results Folder Name")) -> (appended path=w396:path)
        n183 = Concatenate Strings("Target_Value_" ("string"), w391) -> (w392:string)
        n184 = for {
          tunnel: w384 -> [w418] mode=indexing
          tunnel: w396 -> [w417]
          tunnel: w395 -> [w416]
          tunnel: string[] ["Values", "Inputs", "HW Velocity", "Resuduals"] -> [w414] mode=indexing
          tunnel: w392 -> [w413]
          w409 = "_" ("string")
          n185 = Concatenate Strings(w416, w409, w414, w409, w413, ".xls" ("string")) -> (w410:string)
          n186 = Build Path(base path=w417, name or relative path=w410) -> (appended path=w408:path)
          n187 = call <vilib>:"Check if File or Folder Exists.vi"("path"=w408) -> ("dup path"=w411:path)  [unwired: 8 in, 2 out]
          n188 = call "Create_directory_path.vi"("Path name"=w411) -> ("Path name Out"=w415:path)  [unwired: 1 in, 1 out]
          n189 = call-poly <vilib>:"Write To Spreadsheet File.vi"("append to file? (new file:F)"=TRUE, "2D data"=w418, "file path (dialog if empty)"=w415) -> ()  [unwired: 5 in, 1 out]
        }
      }
    }
  }
